vi "Add Subscriber.vi"(8 "error in (no error)":errorcluster, 10 "New FIFO Instance Config":T1, 11 "CIF_Fifo_U8 in":refnum<class "CIF_Fifo_L2Enet_Multi.lvclass">) -> (0 "error out":errorcluster, 2 "New Publisher":string, 3 "CIF_Fifo_U8 out":refnum<class "CIF_Fifo_L2Enet_Multi.lvclass">)   [LabVIEW 2021, in "CIF_Fifo_L2Enet_Multi.lvclass"]
uses:
  CIF_Fifo_L2Enet_Multi.lvclass
  D:/dev/Packages/Channel_Manager/src/CIFChannels/CIFChannels.lvclass
  ChannelCommon/typedef/New FIFO Instance Configuration.ctl
  CIF_Fifo_L2Enet_Multi.lvclass/CIF_Fifo_L2Enet_Multi.ctl
  CIFChannels/Typedef/Direction.ctl
  FIFO_U8/CIF_NIChn_Fifo_U8.lvclass
  CIFChannels/CIFChannels.lvclass
  ChannelCommon/ChannelCommon.lvlib
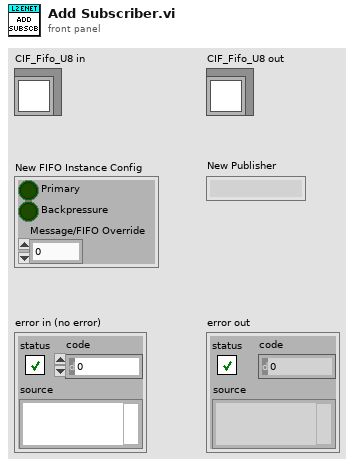
[diagram p1: front panel]
types:
  T1 = typedef "ChannelCommon.lvlib/New FIFO Instance Configuration.ctl" = cluster{"Primary":bool, "Backpressure":bool, "Message/FIFO Override":u32}
  T2 = typedef "CIFChannels.lvclass/Direction.ctl" = enum16{"Publisher", "Subscriber"}
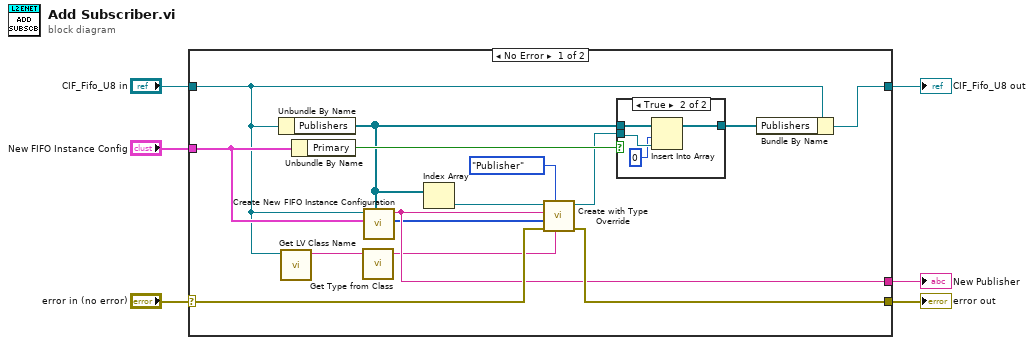
[diagram p0: block diagram]
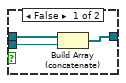
[diagram p2: hidden frame]
diagram:
  n1 = case shown="No Error" "error in (no error)" {
    selector: "error in (no error)" -> [w13 w30]
    tunnel: [w15 w30] -> w5
    tunnel: [w17 w29] -> w3
    tunnel: "CIF_Fifo_U8 in" -> [w9 w29]
    tunnel: "New FIFO Instance Config" -> [w14 _]
    tunnel: [w12 _] -> w1
    frame No Error {
      n2 = Unbundle By Name(w9) -> ("Publishers"=w10:refnum<class "CIF_NIChn_Fifo_U8.lvclass">[])
      n3 = call <vilib>:"Get LV Class Name.vi"("object"=w9) -> ("class name"=w8:string)  [unwired: 9 in, 1 out]
      n4 = Unbundle By Name(w14) -> ("Primary"=w19:bool)
      n5 = call "Get Type from Class.vi"("Class"=w8) -> ("Channel Type"=w7:string)  [unwired: 4 in]
      n6 = call "Create New FIFO Instance Configuration.vi"("Publisher Array in"=w10, "New FIFO Instance Config"=w14, "CIFChannels.lvclass"=w9) -> ("Flattened FIFO Config"=w11:u8[], "New Publisher"=w12:string)  [unwired: 7 in]
      n7 = Index Array(array=w10) -> (element=w21:refnum<class "CIF_NIChn_Fifo_U8.lvclass">)  [unwired: 1 in]
      n8 = call "Create with Type Override.vi"("Type Override"=w7, "Direction"=Direction."Publisher", "error in (no error)"=w13, "Custom Config Data"=w11, "Name"=w12, "CIFFIFO in"=w21) -> ("error out"=w15:errorcluster, "CIFFIFO out"=w16:refnum<class "CIF_NIChn_Fifo_U8.lvclass">)  [unwired: 4 in]
      n9 = case shown="True" w19 {
        tunnel: w10 -> [w24 w28]
        tunnel: [w23 w25] -> w18
        tunnel: w16 -> [w22 w27]
        frame False {
          n10 = Build Array (concatenate)(w24, w22) -> (w23:refnum<class "CIF_NIChn_Fifo_U8.lvclass">[])
        }
        frame True {
          n11 = Insert Into Array(array=w28, index=0, new element=w27) -> (w25:refnum<class "CIF_NIChn_Fifo_U8.lvclass">[])
        }
      }
      n12 = Bundle By Name(cluster=w9, "Publishers"=w18) -> (w17:refnum<class "CIF_Fifo_L2Enet_Multi.lvclass">)
    }
    frame Error {
    }
  }
  "error out" <- w5
  "CIF_Fifo_U8 out" <- w3
  "New Publisher" <- w1
